vi "Backup INI Data.vi"(8 "error in":errorcluster) -> (0 "error out":errorcluster, 2 "INI Data Backup":T1)   [LabVIEW 2020, in "Editor Position.lvclass"]
doc: "Back up the INI data in order to restore it after unit testing."
uses:
  Editor Position.lvclass
  Editor Position.lvclass/Editor Position.ctl
  <resource>/dialog/lvconfig.llb/LV Config Read String.vi
  <resource>/dialog/lvconfig.llb/LV Config Read Boolean.vi
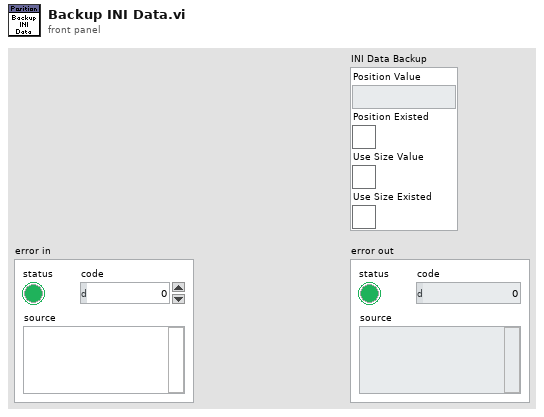
[diagram p1: front panel]
types:
  T1 = cluster{"Position Value":string, "Position Existed":bool, "Use Size Value":bool, "Use Size Existed":bool}
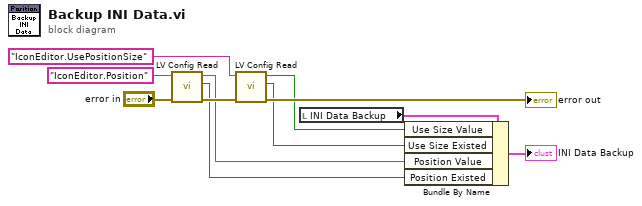
[diagram p0: block diagram]
diagram:
  n1 = call-poly <resource>:"LV Config Read.vi"("error in"="error in", "key"="IconEditor.Position") -> ("error out"=w11:errorcluster, "found?"=w2:bool, "value"=w3:string)  [unwired: 3 in]
  n2 = call-poly <resource>:"LV Config Read.vi"("error in"=w11, "key"="IconEditor.UsePositionSize") -> ("error out"=→"error out":errorcluster, "found?"=w4:bool, "value"=w5:bool)  [unwired: 3 in]
  n3 = local read "INI Data Backup"() -> (w6:T1)
  n4 = Bundle By Name(cluster=w6, "Use Size Value"=w5, "Use Size Existed"=w4, "Position Value"=w3, "Position Existed"=w2) -> (→"INI Data Backup":T1)
